vi "Detect Rising Edge.vi"(7 "signal":bool) -> (8 "edge detected":bool)   [LabVIEW 2013, in "Engine Simulation Toolkit.lvlib"]
doc: "Detects a transition from FALSE to TRUE on the input signal. \n\n<B>Input Parameters</B>\n\n<B>signal</B> specifies the signal in which to detect a FALSE to TRUE transition.\n\n<B>Output Parameters</B>\n\n<B>edge detected</B> indicates whether a FALSE to TRUE transition is detected on the input signal."
uses:
  Engine Simulation Toolkit.lvlib
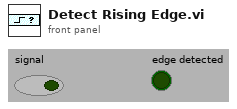
[diagram p1: front panel]
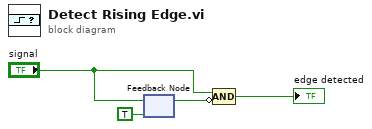
[diagram p0: block diagram]
diagram:
  n1 = feedback-in #1("signal") -> ()
  n2 = feedback #1(TRUE) -> (w3:bool)
  n3 = Compound Arithmetic op=AND("signal", invert w3) -> (→"edge detected":bool)
